vi "Show Child.vi"(8 "error in (no error)":errorcluster, 10 "hwnd":u32, 11 "LV MDI in":refnum<class "LV MDI.lvclass">) -> (0 "error out":errorcluster, 3 "LV MDI out":refnum<class "LV MDI.lvclass">)   [LabVIEW 2016, in "LV MDI.lvclass"]
uses:
  LV MDI.lvclass
  user32.dll
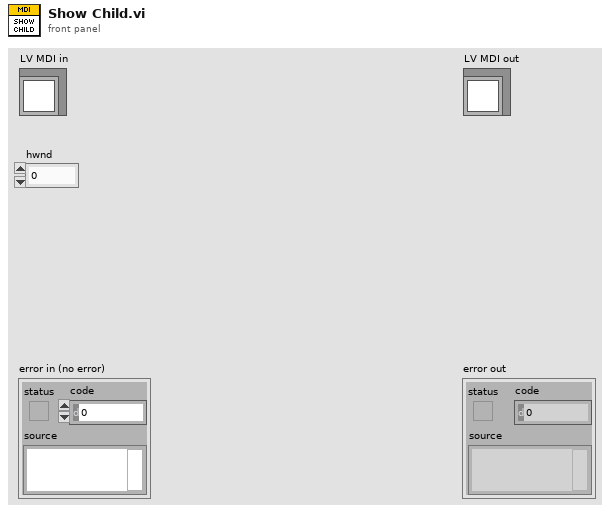
[diagram p1: front panel]
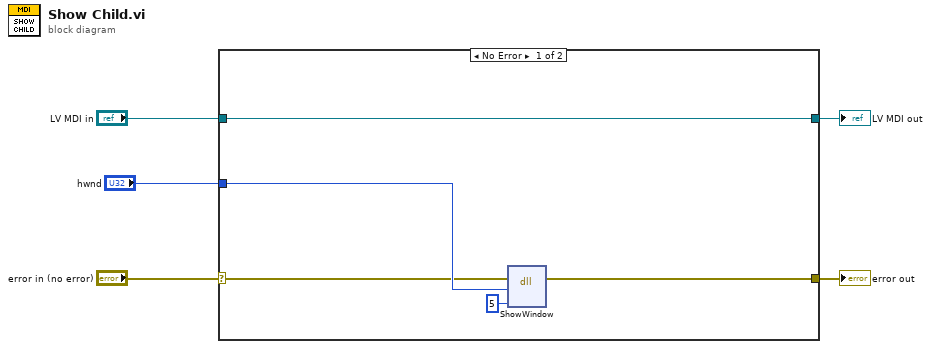
[diagram p0: block diagram]
diagram:
  n1 = case shown="No Error" "error in (no error)" {
    selector: "error in (no error)" -> [w7 w12]
    tunnel: [w6 w12] -> w4
    tunnel: [w10 w11] -> w2
    tunnel: "LV MDI in" -> [w10 w11]
    tunnel: "hwnd" -> [w8 _]
    frame No Error {
      n2 = dll-call lib="user32.dll" fn="ShowWindow"(error in=w7, "hwnd"=w8, "nCmdShow"=u32 5) -> (error out=w6:errorcluster)  [unwired: 5 in, 1 out]
    }
    frame Error {
    }
  }
  "error out" <- w4
  "LV MDI out" <- w2
